vi "clear Session Data.vi"(0 "OBJ - Measurement Session in":refnum<class "Config Data.lvclass">, 11 "error in":errorcluster) -> (4 "OBJ - Measurement Session out":refnum<class "Config Data.lvclass">, 15 "error out":errorcluster)   [LabVIEW 2014, in "Config Data.lvclass"]
doc: "OVERRIDE VI\nPlaceholder for decendant classes to clear session information and close references."
uses:
  Config Data.lvclass
  Config Data.lvclass/Config Data.ctl
  <vilib>/Utility/config.llb/NI_LVConfig.lvlib
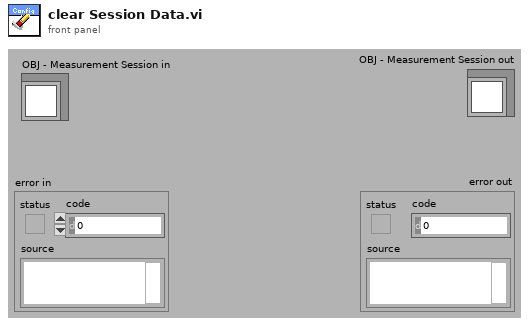
[diagram p1: front panel]
types:
  T1 = typedef "NI_LVConfig.lvlib/Config Data RefNum.ctl" = refnum<k1>
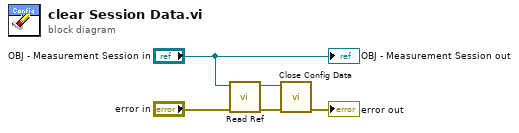
[diagram p0: block diagram]
diagram:
  n1 = call "Read Ref.vi"("error in"="error in", "Config Data in"="OBJ - Measurement Session in") -> ("error out"=w4:errorcluster, "config data"=w5:T1)  [unwired: 7 in, 1 out]
  n2 = call <vilib>:"Close Config Data.vi"("error in (no error)"=w4, "refnum"=w5) -> ("error out"=→"error out":errorcluster)  [unwired: 8 in, 1 out]
  "OBJ - Measurement Session out" <- "OBJ - Measurement Session in"
